vi "type.get.vi"(8 "error in (no error)":errorcluster, 11 "asset in":refnum<class "asset.lvclass">) -> (0 "error out":errorcluster, 2 "type":refnum<class "type.lvclass">, 3 "asset out":refnum<class "asset.lvclass">)   [LabVIEW 2020, in "asset.lvclass"]
uses:
  asset.lvclass
  asset.lvclass/asset.ctl
  Nominal Client/Nominal Client.lvclass
  type/type.lvclass
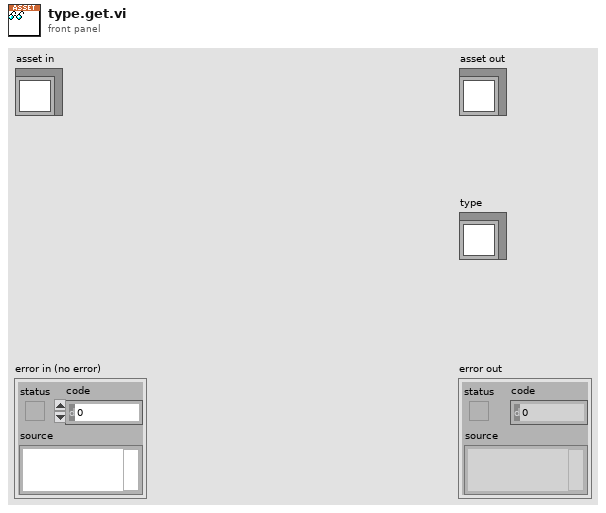
[diagram p1: front panel]
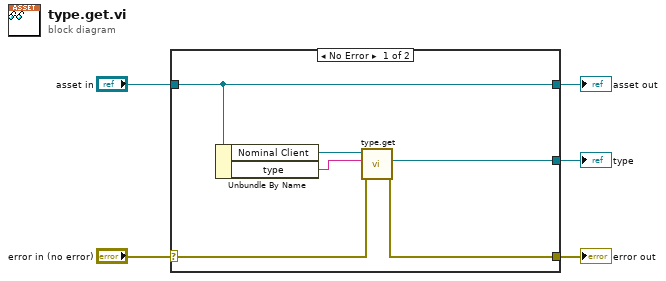
[diagram p0: block diagram]
diagram:
  n1 = case shown="No Error" "error in (no error)" {
    selector: "error in (no error)" -> [w6 w12]
    tunnel: [w7 w12] -> w4
    tunnel: [w11 w13] -> w2
    tunnel: "asset in" -> [w11 w13]
    tunnel: [w8 _] -> w1
    frame No Error {
      n2 = Unbundle By Name(w11) -> ("Nominal Client"=w10:refnum<class "Nominal Client.lvclass">, "type"=w9:string)
      n3 = call "type.get.vi"("error in"=w6, "Type RID"=w9, "Nominal Client in"=w10) -> ("error out"=w7:errorcluster, "type"=w8:refnum<class "type.lvclass">)  [unwired: 6 in, 1 out]
    }
    frame Error {
    }
  }
  "error out" <- w4
  "asset out" <- w2
  "type" <- w1
